vi "StringToTimeStamp.vi"(11 "タイムスタンプ(String)":string) -> (3 "タイムスタンプ(Data)":timestamp)   [LabVIEW 2014]
uses:
  <vilib>/Utility/miscctls.llb/LVDateTimeRec.ctl
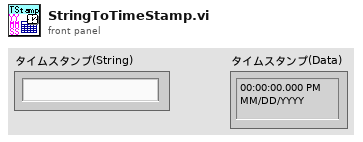
[diagram p1: front panel]
types:
  T1 = typedef "LVDateTimeRec.ctl" = cluster{"fractional second":dbl, "second":i32, "minute":i32, "hour":i32, "day of month":i32, "month":i32, "year":i32, "day of week":i32, "day of year":i32, "DST":i32}
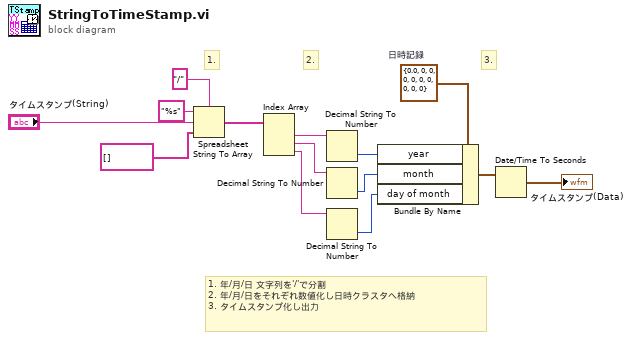
[diagram p0: block diagram]
diagram:
  w5 = T1 {"fractional second"=0.0, "second"=0, "minute"=0, "hour"=0, "day of month"=0, "month"=0, "year"=0, "day of week"=0, "day of year"=0, "DST"=0}  # 日時記録
  # "1. 年/月/日 文字列を'/'で分割\n2. 年/月/日をそれぞれ数値化し日時クラスタへ格納\n3. タイムスタンプ化し出力"
  # "3."
  # "2."
  # "1."
  n1 = Spreadsheet String To Array(delimiter (Tab)="/" ("デリミタ（タブ）"), format string="%s" ("形式文字列"), spreadsheet string="タイムスタンプ(String)", array type (2D Dbl)=string[] []) -> (array=w9:string[])
  n2 = Index Array(array=w9) -> (element #1=w8:string, element #2=w7:string, element #3=w6:string)  [unwired: 3 in]
  n3 = Decimal String To Number(string=w8) -> (number=w4:i32)  [unwired: 2 in, 1 out]
  n4 = Decimal String To Number(string=w7) -> (number=w3:i32)  [unwired: 2 in, 1 out]
  n5 = Decimal String To Number(string=w6) -> (number=w2:i32)  [unwired: 2 in, 1 out]
  n6 = Bundle By Name(cluster=w5, "year"=w4, "month"=w3, "day of month"=w2) -> (w1:T1)
  n7 = Date/Time To Seconds(2:w1) -> (0:→"タイムスタンプ(Data)":timestamp)  [unwired: 1 in]
